vi "Teleop LED Control.vi"(9 "D-Pad":T2, 11 "Axes":T1) -> ()   [LabVIEW 2017]
uses:
  Common Code/Gamepads/D-Pad.ctl
  Common Code/Gamepads/Axes Cluster.ctl
  Robot Global Data.vi
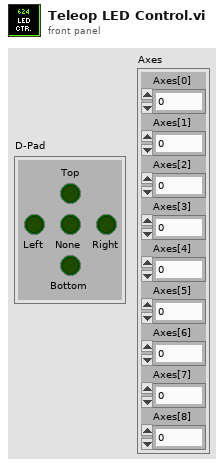
[diagram p1: front panel]
types:
  T1 = typedef "Axes Cluster.ctl" = cluster{"Axes[0]":dbl, "Axes[1]":dbl, "Axes[2]":dbl, "Axes[3]":dbl, "Axes[4]":dbl, "Axes[5]":dbl, "Axes[6]":dbl, "Axes[7]":dbl, "Axes[8]":dbl}
  T2 = typedef "D-Pad.ctl" = cluster{"Top":bool, "Bottom":bool, "None":bool, "Right":bool, "Left":bool}
  T3 = typedef "LED Command Cluster.ctl" = cluster{"Driver RED":bool, "Driver BLUE":bool, "Saboi":bool}
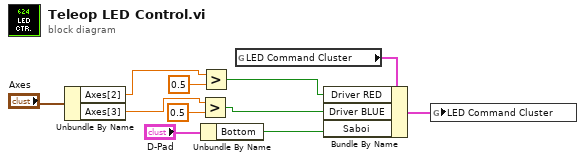
[diagram p0: block diagram]
diagram:
  n1 = Unbundle By Name("Axes") -> ("Axes[2]"=w4:dbl, "Axes[3]"=w3:dbl)
  n2 = Greater?(x=w3, y=0.5) -> (0:w2:bool)
  n3 = Greater?(x=w4, y=0.5) -> (0:w1:bool)
  n4 = Unbundle By Name("D-Pad") -> ("Bottom"=w8:bool)
  n5 = global read "Robot Global Data.vi" "LED Command Cluster"() -> (w11:T3)
  n6 = Bundle By Name(cluster=w11, "Driver RED"=w1, "Driver BLUE"=w2, "Saboi"=w8) -> (w10:T3)
  n7 = global write "Robot Global Data.vi" "LED Command Cluster"(w10) -> ()
